vi "Communication Trigger.vi"(6 "Source Type (0:Data)":u16(ring) items=["Data", "Clock", "Recovered"], 8 "Bit Rate (1.544E6Mb/s)":dbl=1544000.0, 9 "Standard (0:ATAG1)":u16(ring) items=["ATAG1", "ATAG2", "ATAG3", "Clock Coax", "Clock Symmetrical", "D1", "D2", "DS0 Contra", "DS0 Double", "DS0 Single", "DS0Timing", "DS1", "DS1A", "DS1C", "DS2", "DS2RATE Symmetrical", "DS2RATE Coax", "RATE32Mbit", "RATE97Mbit", "DS3", "DS4NA", "E1", "E2", "E3", "E4", "STS1", "STS3", "STM1E", "FC133", "FC266", "FC531", "FC1063", "FC2125", "FC4250", "OC1", "OC3", "OC12", "OC48", "OC48_FEC", "STM1E", "ENET100", "ENET1250", "ENETXAUI", "INF2_5G", "FST", "HST", "FW1394BS400B", "FW1394BS1600B", "RIO_500M", "RIO_750M", "RIO_1G", "RIO_1_5G", "RIO_2G", "RIO_SERIAL_1G", "RIO_SERIAL_2G", "RIO_SERIAL_3G", "SAS1_5", "SAS3_0", "SFI5_2", "STM0_HDBX", "STM0_CMI", "RATE32Mbit", "RATE97Mbit", "SFI5_3", "VSROC192", "TFI5_2", "TFI5_3", "PCIEXPRESS", "VIDEO270", "VIDEO360", "Custom", "VIDEO292M"], 10 "Coding (0:NRZ)":u16(ring) items=["NRZ", "MLT3", "AMI", "HDB3", "B3ZS", "B6ZS", "B8ZS", "CMI"], 11 "Source (0:Channel1)":u16(ring) items=["Channel 1", "Channel 2", "Channel 3", "Channel 4"]) -> (1 "Output String":string)   [LabVIEW 2011, in "Tektronix 7000 Series.lvlib"]
doc: "Configures the common settings for the Communication Trigger."
uses:
  Tektronix 7000 Series.lvlib
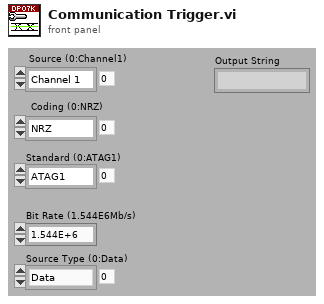
[diagram p1: front panel]
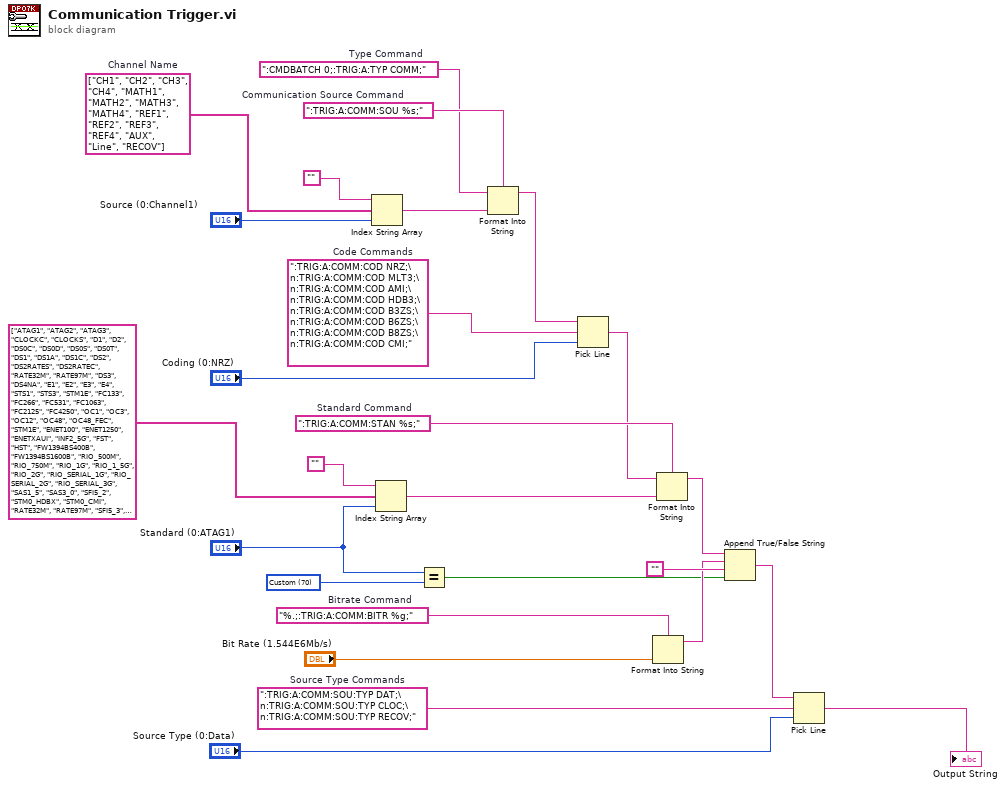
[diagram p0: block diagram]
diagram:
  w24 = ":TRIG:A:COMM:SOU:TYP DAT;\n:TRIG:A:COMM:SOU:TYP CLOC;\n:TRIG:A:COMM:SOU:TYP RECOV;"  # Source Type Commands
  w21 = "%.;:TRIG:A:COMM:BITR %g;"  # Bitrate Command
  w17 = u16 70 items=["ATAG1"=0, "ATAG2"=1, "ATAG3"=2, "D1"=5, "D2"=6, "RATE32Mbit"=17, "RATE97Mbit"=18, "STS1"=25, "STS3"=26, "STM1E"=27, "FC133"=28, "FC266"=29, "FC531"=30, "FC1063"=31, "FC2125"=32, "FC4250"=33, "OC1"=34, "OC3"=35, "OC12"=36, "OC48"=37, "OC48_FEC"=38, "STM1E"=39, "ENET100"=40, "ENET1250"=41, "ENETXAUI"=42, "INF2_5G"=43, "FST"=44, "HST"=45, "FW1394BS400B"=46, "FW1394BS1600B"=47, "RIO_500M"=48, "RIO_750M"=49, "RIO_1G"=50, "RIO_1_5G"=51, "RIO_2G"=52, "RIO_SERIAL_1G"=53, "RIO_SERIAL_2G"=54, "RIO_SERIAL_3G"=55, "SAS1_5"=56, "SAS3_0"=57, "SFI5_2"=58, "STM0_HDBX"=59, "STM0_CMI"=60, "RATE32Mbit"=61, "RATE97Mbit"=62, "SFI5_3"=63, "VSROC192"=64, "TFI5_2"=65, "TFI5_3"=66, "PCIEXPRESS"=67, "VIDEO270"=68, "VIDEO360"=69, "Custom"=70] ("Standard (0:ATAG1)")
  w16 = ":TRIG:A:COMM:STAN %s;"  # Standard Command
  w13 = ":TRIG:A:COMM:COD NRZ;\n:TRIG:A:COMM:COD MLT3;\n:TRIG:A:COMM:COD AMI;\n:TRIG:A:COMM:COD HDB3;\n:TRIG:A:COMM:COD B3ZS;\n:TRIG:A:COMM:COD B6ZS;\n:TRIG:A:COMM:COD B8ZS;\n:TRIG:A:COMM:COD CMI;"  # Code Commands
  w10 = ":TRIG:A:COMM:SOU %s;"  # Communication Source Command
  w9 = ":CMDBATCH 0;:TRIG:A:TYP COMM;"  # Type Command
  w8 = string[] ["CH1", "CH2", "CH3", "CH4", "MATH1", "MATH2", "MATH3", "MATH4", "REF1", "REF2", "REF3", "REF4", "AUX", "Line", "RECOV"]  # Channel Name
  n1 = Index String Array(1:"Source (0:Channel1)", 2:w8, 3:"" ("Empty String Constant")) -> (0:w11:string)
  n2 = Index String Array(1:"Standard (0:ATAG1)", 2:string[] ["ATAG1", "ATAG2", "ATAG3", "CLOCKC", "CLOCKS", "D1", "D2", "DS0C", "DS0D", "DS0S", "DS0T", "DS1", "DS1A", "DS1C", "DS2", "DS2RATES", "DS2RATEC", "RATE32M", "RATE97M", "DS3", "DS4NA", "E1", "E2", "E3", "E4", "STS1", "STS3", "STM1E", "FC133", "FC266", "FC531", "FC1063", "FC2125", "FC4250", "OC1", "OC3", "OC12", "OC48", "OC48_FEC", "STM1E", "ENET100", "ENET1250", "ENETXAUI", "INF2_5G", "FST", "HST", "FW1394BS400B", "FW1394BS1600B", "RIO_500M", "RIO_750M", "RIO_1G", "RIO_1_5G", "RIO_2G", "RIO_SERIAL_1G", "RIO_SERIAL_2G", "RIO_SERIAL_3G", "SAS1_5", "SAS3_0", "SFI5_2", "STM0_HDBX", "STM0_CMI", "RATE32M", "RATE97M", "SFI5_3", "VSROC192", "TFI5_2", "TFI5_3", "PCIEXPRESS", "VIDEO270", "VIDEO360", "CUST", "VIDEO292M"], 3:"" ("Empty String Constant")) -> (0:w14:string)
  n3 = Equal?(x="Standard (0:ATAG1)", y=w17) -> (x = y?=w18:bool)
  n4 = Format Into String(format string=w10, initial string=w9, w11) -> (resulting string=w12:string)  [unwired: 1 in, 1 out]
  n5 = Pick Line(string ("")=w12, multi-line string=w13, line index="Coding (0:NRZ)") -> (output string=w15:string)
  n6 = Format Into String(format string=w21, "Bit Rate (1.544E6Mb/s)") -> (resulting string=w22:string)  [unwired: 2 in, 1 out]
  n7 = Format Into String(format string=w16, initial string=w15, w14) -> (resulting string=w19:string)  [unwired: 1 in, 1 out]
  n8 = Append True/False String(1:w18, 2:"" ("Empty String Constant"), 3:w22, 4:w19) -> (0:w25:string)
  n9 = Pick Line(string ("")=w25, multi-line string=w24, line index="Source Type (0:Data)") -> (output string=→"Output String":string)
